vi "GetSRsbyStatus.vi"(6 "Period":T1={"Start Date"=timestamp(-113047311.23669147 s since 1904-01-01), "End Date"=timestamp(9354056288.76331 s since 1904-01-01)}, 7 "Statuses":string[](array[string]), 8 "Error In":errorcluster, 11 "Report DVR in":refnum<data-value>) -> (0 "Error Out":errorcluster, 2 "SRs Out":T2[](array[typedef]), 3 "Report DVR out":refnum<data-value>)   [LabVIEW 2018, in "DS_Lib.lvlib" / "SRReportParser.lvlib"]
uses:
  SRReportParser.lvlib
  TypeDefs/InWorkSR_Data.ctl
  Modules/Private Controls/Report Data Cluster.ctl
  Modules/Private Controls/Data Raw.ctl
  Modules/Data Operations.lvlib
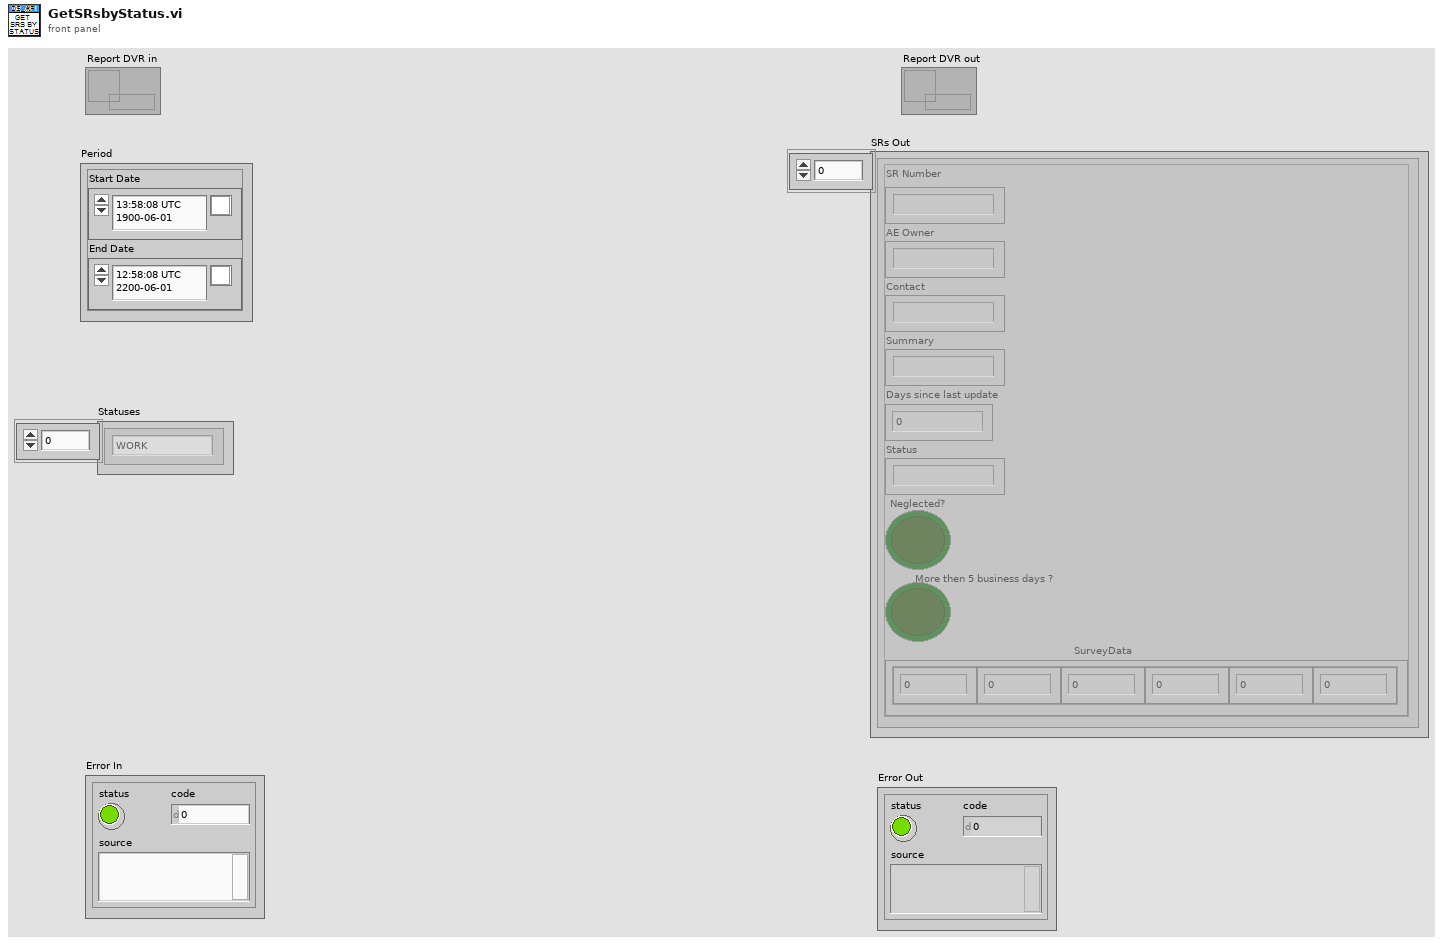
[diagram p1: front panel]
types:
  T1 = cluster{"Start Date":timestamp, "End Date":timestamp}
  T2 = typedef "DS_Lib.lvlib/SRReportParser.lvlib/InWorkSR_Data.ctl" = cluster{"SR Number":string, "AE Owner":string, "Contact":string, "Summary":string, "Days since last update":dbl, "Status":string, "Neglected?":bool, "More then 5 business days ?":bool, "SurveyData":cluster{"Resolution Time":dbl, "Total Satisfaction":dbl, "Response Time":dbl, "Courtesy":dbl, "Problem Solved":dbl, "Level of effort":dbl}}
  T3 = typedef "Data Operations.lvlib/Report Data Cluster.ctl" = cluster{"Headers":cluster{"Start Date":timestamp, "End Date":timestamp, "SR Status String":string[], "AE Owner String":string[]}, "Data":T4[]}
  T4 = typedef "Data Operations.lvlib/Data Raw.ctl" = cluster{"SR Number":string, "Status":string, "Summary":string, "AE Owner":string, "AE Group":string, "Contact":string, "SurveyData":cluster{"Resolution Time":dbl, "Total Satisfaction":dbl, "Response Time":dbl, "Courtesy":dbl, "Problem Solved":dbl, "Level of effort":dbl}, "Time Data":cluster{"Last Update Date":timestamp, "Creation Date":timestamp, "Creation week":i16, "Last Update Week":i16, "Creation Year":i16}}
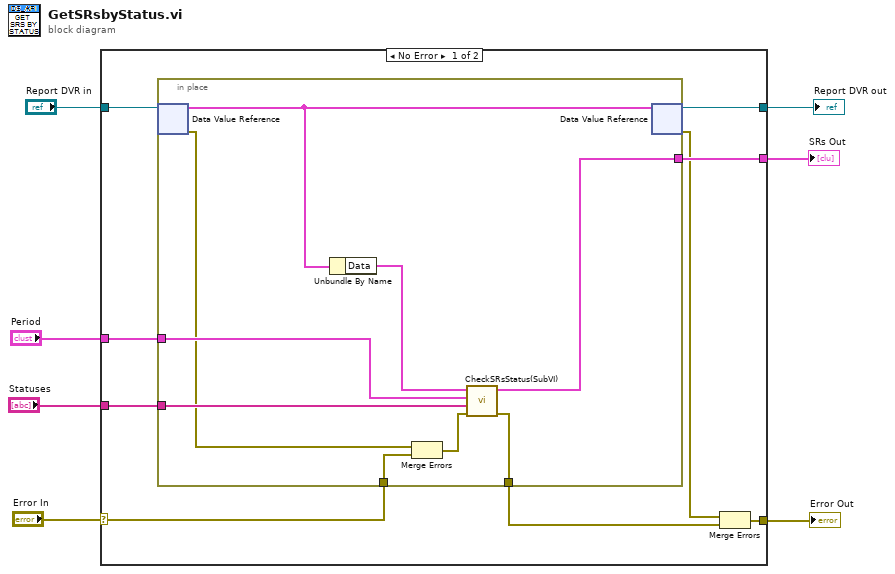
[diagram p0: block diagram]
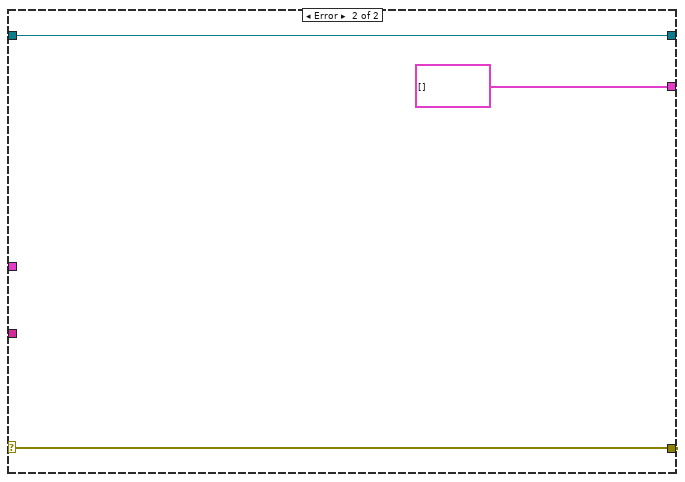
[diagram p2: hidden frame]
diagram:
  n1 = case shown="No Error" "Error In" {
    selector: "Error In" -> [w11 w27]
    tunnel: "Report DVR in" -> [w16 w28]
    tunnel: [w8 w27] -> w6
    tunnel: [w15 w28] -> w1
    tunnel: "Statuses" -> [w14 _]
    tunnel: [w12 T2[] []] -> w4
    tunnel: "Period" -> [w13 _]
    frame No Error {
      n2 = in-place {
        in-place-border: w14 -> [w24]
        in-place-border: w13 -> [w23]
        in-place-border: [w21] -> w12
        in-place-border: w11 -> [w19]
        in-place-border: [w22] -> w9
        n3 = in-place-dvr #1(w16) -> (w25:T3, w18:errorcluster)
        n4 = Unbundle By Name(w25) -> ("Data"=w20:T4[])
        n5 = Merge Errors(w18, w19) -> (w17:errorcluster)
        n6 = call "CheckSRsStatus(SubVI).vi"("Error In"=w17, "Statuses"=w24, "Period"=w23, "Report Data In"=w20) -> ("Error Out"=w22:errorcluster, "SR Data Out"=w21:T2[])  [unwired: 6 in]
        n7 = in-place-dvr #1(w25) -> (w15:refnum<data-value>, w10:errorcluster)
      }
      n8 = Merge Errors(w10, w9) -> (w8:errorcluster)
    }
    frame Error {
    }
  }
  "Error Out" <- w6
  "SRs Out" <- w4
  "Report DVR out" <- w1
